vi "Write supported targets.vi"(8 "error in":errorcluster, 10 "supported targets":T1[](array[typedef]), 11 "decideprojectfeatures in":refnum<class "DecideModuleFeatures.lvclass">) -> (0 "error out":errorcluster, 3 "decideprojectfeatures out":refnum<class "DecideModuleFeatures.lvclass">)   [LabVIEW 2013, in "DecideModuleFeatures.lvclass"]
uses:
  DecideModuleFeatures.lvclass
  root configuration/Target Types.ctl
  DecideModuleFeatures.lvclass/DecideModuleFeatures.ctl
  root configuration/TBM configuration.lvclass
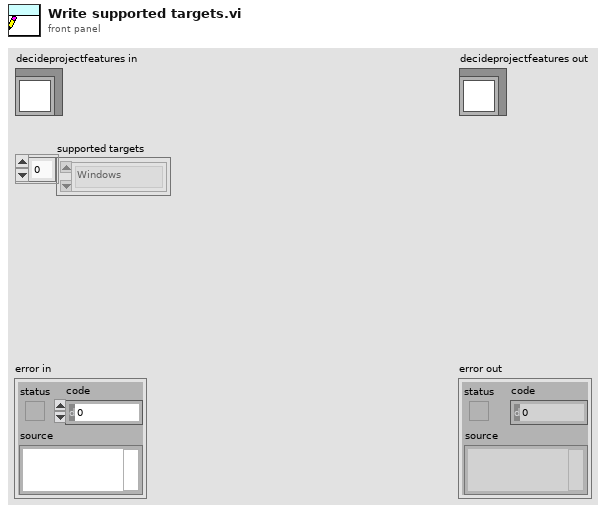
[diagram p1: front panel]
types:
  T1 = typedef "TBM configuration.lvclass/Target Types.ctl" = enum16{"Windows", "Mac", "Linux", "Linux RT ARM", "VxWorks", "Pharlap", "Other", "Linux RT x64"}
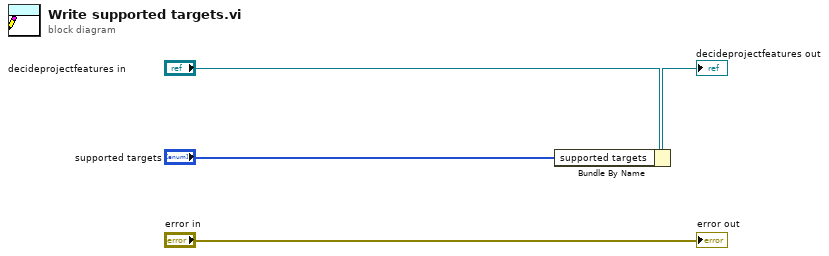
[diagram p0: block diagram]
diagram:
  n1 = Bundle By Name(cluster="decideprojectfeatures in", "supported targets"="supported targets") -> (→"decideprojectfeatures out":refnum<class "DecideModuleFeatures.lvclass">)
  "error out" <- "error in"
